vi "activate.vi"(0 "SEDSpectrometer in":refnum<class "FiberSpectrograph.lvclass">, 5 "DeviceId":u8[](array[numeric]), 11 "error in (no error)":errorcluster) -> (4 "SEDSpectrometer out":refnum<class "FiberSpectrograph.lvclass">, 6 "Device handle":i32, 8 "Activation Error":bool, 10 "DeviceId":u8[](array[numeric]), 15 "error out":errorcluster)   [LabVIEW 2016, in "FiberSpectrograph.lvclass"]
uses:
  FiberSpectrograph.lvclass
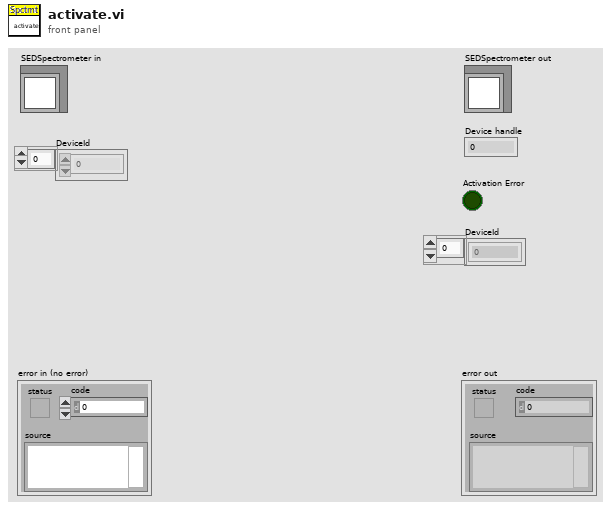
[diagram p1: front panel]
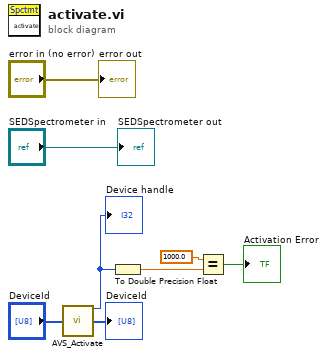
[diagram p0: block diagram]
diagram:
  n1 = call "AVS_Activate.vi"("a_pDeviceId"="DeviceId") -> ("Output Value"=w2:i32, "a_pDeviceId"=→"DeviceId":u8[])  [unwired: 13 in]
  "Device handle" <- w2
  n2 = To Double Precision Float(number=w2) -> (double precision float=w1:dbl)
  n3 = Equal?(x=1000.0, y=w1) -> (x = y?=→"Activation Error":bool)
  "error out" <- "error in (no error)"
  "SEDSpectrometer out" <- "SEDSpectrometer in"
